vi "Read Quantum Desing Configuration.vi"(8 "error in (no error)":errorcluster, 11 "Quantum Design Driver in":refnum<class "Quantum Design Driver.lvclass">) -> (0 "error out":errorcluster, 2 "Quantum Desing Configuration":T1={"Address"="127.0.0.1", "Instrument type"=0, "Remote"=FALSE, "Measurements"=[enum."Temperature"]} {"Instrument type" items=["PPMS", "VersaLab", "DynaCool", "SVSM"]}, 3 "Quantum Design Driver out":refnum<class "Quantum Design Driver.lvclass">)   [LabVIEW 2021, in "Quantum Design Driver.lvclass"]
uses:
  Quantum Design Driver.lvclass
  C:/GitHub/NHMFL_Core/Libraries/Instruments/Instrument Driver/Instrument Driver.lvclass
  Quantum Desing Configuration.ctl
  Instrument Driver/Read User configuration.vi
  Quantum Design Driver.lvclass/Quantum Design Driver.ctl
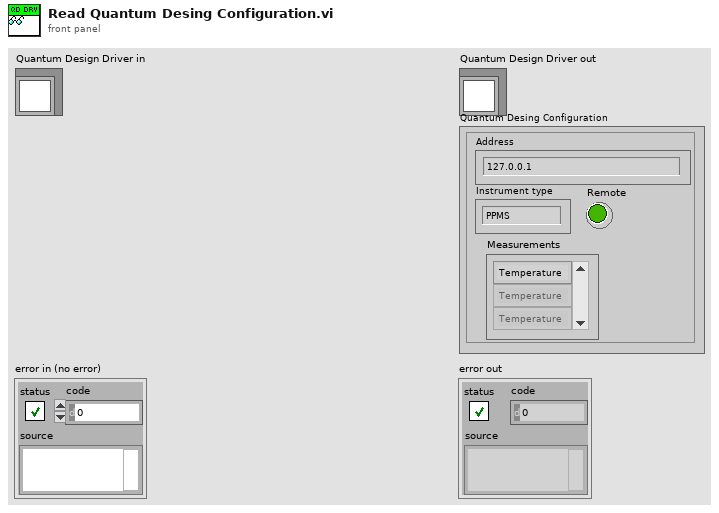
[diagram p1: front panel]
types:
  T1 = typedef "Quantum Desing Configuration.ctl" = cluster{"Address":string, "Instrument type":u16, "Remote":bool, "Measurements":enum16{"Temperature", "Field", "Position"}[]}
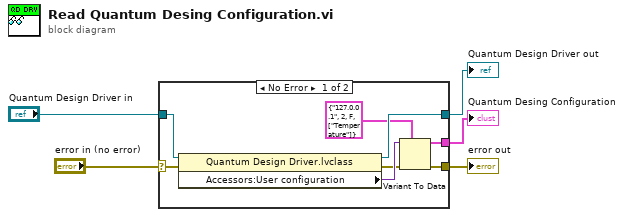
[diagram p0: block diagram]
diagram:
  n1 = case shown="No Error" "error in (no error)" {
    selector: "error in (no error)" -> [w13 w14]
    tunnel: [w7 w14] -> w4
    tunnel: [w11 w15] -> w2
    tunnel: "Quantum Design Driver in" -> [w12 w15]
    tunnel: [w6 _] -> w1
    frame No Error {
      n2 = property class="Quantum Design Driver.lvclass"(reference=w12, error in=w13) -> (reference out=w11:refnum<class "Quantum Design Driver.lvclass">, error out=w8:errorcluster, "Accessors:User configuration"=w9:variant)
      n3 = Variant To Data(error in=w8, type=T1 {"Address"="127.0.0.1", "Instrument type"=2, "Remote"=FALSE, "Measurements"=[enum."Temperature"]} ("Quantum Desing Configuration"), Variant=w9) -> (data=w6:T1, error out=w7:errorcluster)
    }
    frame Error {
    }
  }
  "error out" <- w4
  "Quantum Design Driver out" <- w2
  "Quantum Desing Configuration" <- w1
